vi "翻转矩形（TB）.vi"(10 "Y轴":bool, 11 "矩形":T1) -> (3 "翻转转后矩形":T1)   [LabVIEW 2012, in "Picture Box Tools.lvlib"]
uses:
  RectTB.ctl
  Picture Box Tools.lvlib
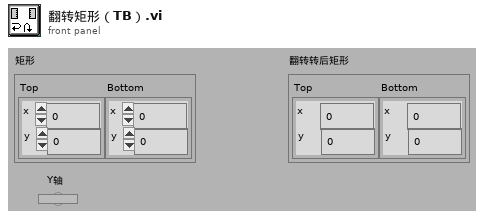
[diagram p1: front panel]
types:
  T1 = typedef "Picture Box Tools.lvlib/RectTB.ctl" = cluster{"Top":cluster{"x":i16, "y":i16}, "Bottom":cluster{"x":i16, "y":i16}}
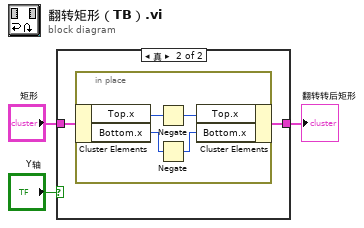
[diagram p0: block diagram]
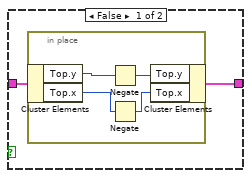
[diagram p2: hidden frame]
diagram:
  n1 = case shown="真" "Y轴" {
    tunnel: "矩形" -> [w5 w11]
    tunnel: [w4 w10] -> w1
    frame False {
      n2 = in-place {
        n3 = in-place-cluster #1(w5) -> ("Top.y"=w9:i16, "Top.x"=w7:i16)
        n4 = Negate(x=w9) -> (-x=w8:i16)
        n5 = Negate(x=w7) -> (-x=w6:i16)
        n6 = in-place-cluster #1("Top.y"=w8, "Top.x"=w6) -> (w4:T1)
      }
    }
    frame True {
      n7 = in-place {
        n8 = in-place-cluster #2(w11) -> ("Top.x"=w15:i16, "Bottom.x"=w13:i16)
        n9 = Negate(x=w15) -> (-x=w14:i16)
        n10 = Negate(x=w13) -> (-x=w12:i16)
        n11 = in-place-cluster #2("Top.x"=w14, "Bottom.x"=w12) -> (w10:T1)
      }
    }
  }
  "翻转转后矩形" <- w1
